vi "RT Main.vi"() -> ()   [LabVIEW 2023]
uses:
  <vilib>/Platform/TimedLoop/XDataNode/timing_clust.ctl
  <vilib>/Platform/TimedLoop/XDataNode/nitl_modes.ctl
  <vilib>/Platform/TimedLoop/XDataNode/wakeup.ctl
  <vilib>/DAQmx/read.llb/DAQmx Read (Analog 1D DBL NChan 1Samp).vi
  <vilib>/DAQmx/create/channels.llb/DAQmx Create Channel (AI-Position-LVDT).vi
  <vilib>/DAQmx/configure/timing.llb/DAQmx Timing (Sample Clock).vi
  <vilib>/DAQmx/miscellaneous.llb/DAQmx Fill In Error Info.vi
  <vilib>/platform/TimedLoop/XDataNode/XDataNode.xnode
  <vilib>/Platform/TimedLoop/XDataNode/XDNodeRunTimeDep.lvlib
panel:
  in  "Stop Button":bool
  in  "SCAS Controller Test Panel":enum32{"LVDT Test Page", "mA Output Test Page"}(tab)
  in  "Physical channels(PXI1Slot3/ai1:0)":tag="PXI1Slot3/ai1:0"
  in  "Voltage Excitation Value":dbl=3.0
  in  "Voltage excitation frequency":dbl=2050.0
  in  "Sensitivity":dbl=1.0
  in  "Samples per channel":i32=1000
  in  "Sample rate":dbl=1000.0 format="%0.2f"
  in  "Voltage excitation wire mode":i32(ring)=5 items=["4-Wire"=4, "5-Wire"=5, "6-Wire"=6]
  in  "Sample mode":i32(ring)=10123 items=["Finite Samples"=10178, "Continuous Samples"=10123, "Hardware Timed Single Point"=12522]
  in  "Sensivity value for calculation":dbl=1.0
  in  "Voltage excitation source":i32(ring)=10200 items=["Internal"=10200, "External"=10167, "None"=10230]
  in  "Sensitivity units":i32(ring)=12506 items=["mVolts/Volt/mMeter"=12506, "mVolts/Volt/0.001 Inch"=12505]
  in  "Units":i32(ring)=10219 items=["Meters"=10219, "Inches"=10379, "From Custom Scale"=10065]
  out "LVDT Output mm":dbl(graph)
  in  "resource name(PXI144::0::INSTR)":string="PXI144::0::INSTR"
  out "id string":string
  in  "Channel Output Number":u32=1
  in  "isolation switch":bool=TRUE
  in  "shorting switch":bool
  in  "Set Value mA":dbl(slide) scale=-24.0..24.0
  out "Get Value mA":dbl
  out "attr mode":u32
  out "error out":errorcluster
  # "Note1: Change Sensivity for adjusting the LVDT Output mm. 4340 reads the LVDT sensor mVolts/Volt/meter."
  # "Note2: Change Sensivity value for calculation if the sensivity is not enough to calculate LVDT Output mm"
  # "Note3: DONT assign 0 value for sensivity and sensivity value for calculation"
  # "Check the pickering card id"
  # "Check the Attr Mode is 3. 3 represents the -24 / +24 mA curret output mode."
  # "Check the isolation switch is \"CLOSE\"(1).(The button default state is \"OPEN\" inside pickering board)"
  # "Check the shorting switch is \"OPEN\"(0).(The button default state is \"OPEN\" inside pickering board)"
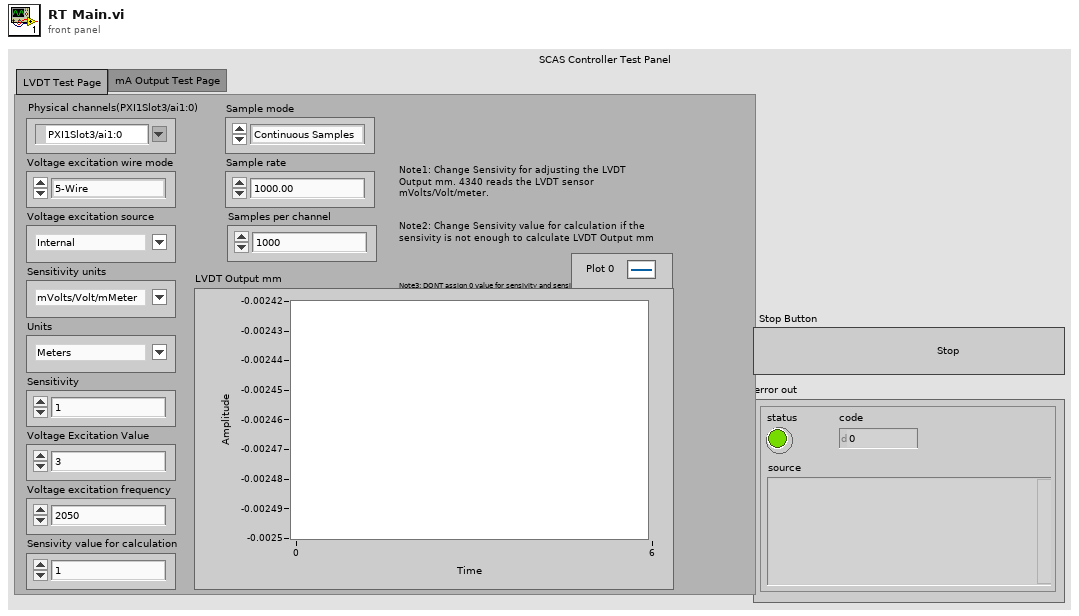
[diagram p1: front panel]
types:
  T1 = typedef "XDNodeRunTimeDep.lvlib/timing_clust.ctl" = cluster{"Expected End [f-1]":u64, "Actual End [f-1]":u64, "Finished Late? [f-1]":bool, "Expected End [i-1]":u64, "Actual End [i-1]":u64, "Finished Late? [i-1]":bool, "Expected Start [i]":u64, "Actual Start [i]":u64, "Expected Start [f]":u64, "Actual Start [f]":u64, "Source Name":string, "Structure Name":string, "Period":i64, "Deadline":i64, "Offset":i64, "Start":i64, "Priority":i32, "Timeout":i32, "Mode":T2, "Wakeup Reason":T3, "Error":errorcluster, "Source Type":string, "Secondary Source Type":string, "Global End Time":u64, "Global Start Time":u64, "Frame Duration":u64, "Iteration Duration":u64, "Assigned CPU":i32, "I/O Scan Engine Mode":u32}
  T2 = typedef "XDNodeRunTimeDep.lvlib/nitl_modes.ctl" = enum32{"No Change", "Process missed periods, maintain original phase", "Discard missed periods, maintain original phase", "Process missed periods, ignore original phase", "Discard missed periods, ignore original phase"}
  T3 = typedef "XDNodeRunTimeDep.lvlib/wakeup.ctl" = enum32{"Normal", "Aborted", "Asynchronous wakeup", "Timing source error", "Timed loop error", "Timeout"}
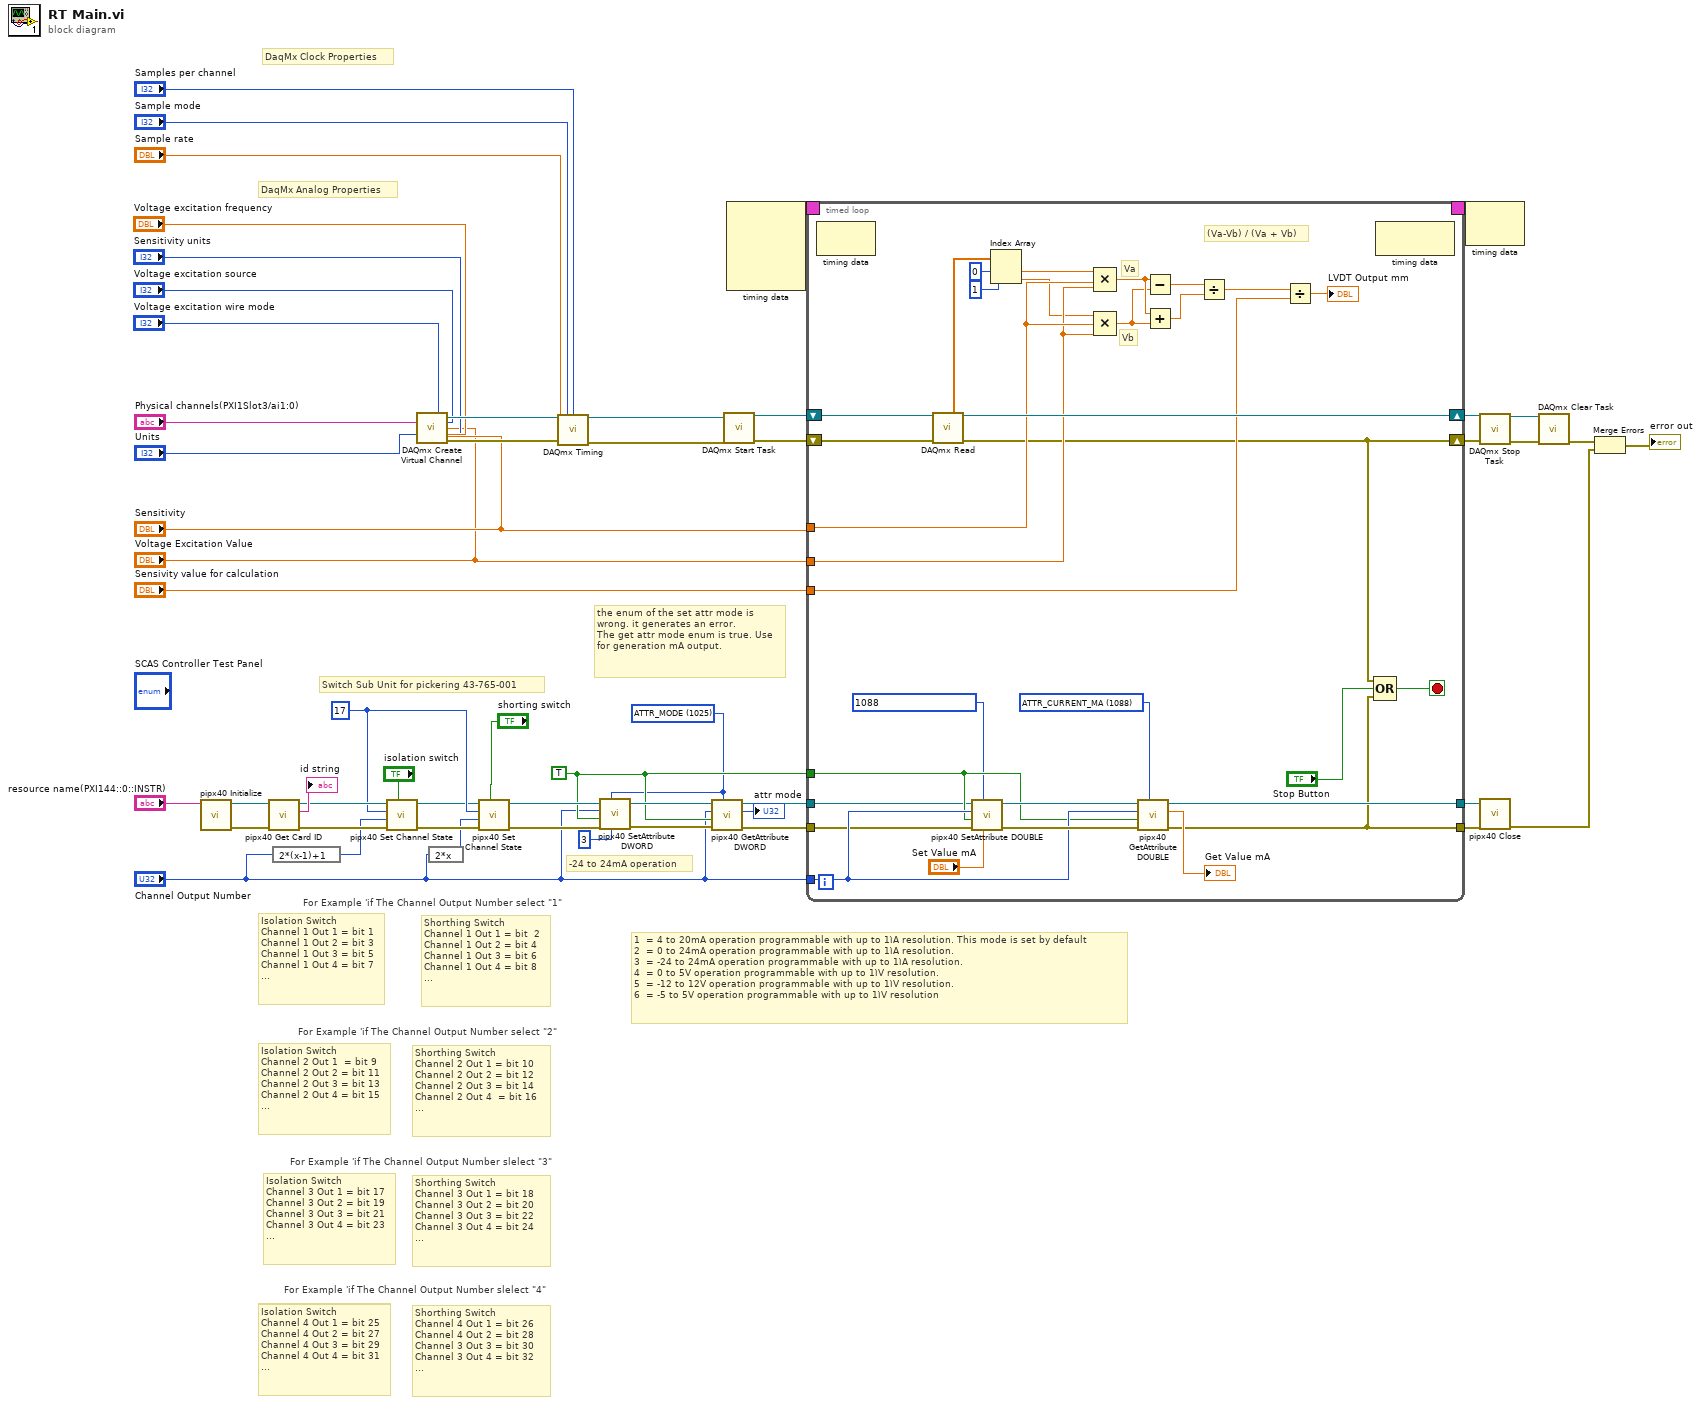
[diagram p0: block diagram]
diagram:
  w6 = u16 1025 items=["ATTR_TYPE"=1024, "ATTR_MODE"=1025, "ATTR_TS_SET_RANGE"=1034, "ATTR_VDT_AUTO_INPUT_ATTEN"=1104, "ATTR_VDT_ABS_POSITION"=1105, "ATTR_VDT_ABS_POSITION_B"=1106, "ATTR_VDT_OUT_GAIN   "=1111, "ATTR_VDT_MANUAL_INPUT_ATTEN"=1112, "ATTR_VDT_MODE"=1113, "ATTR_VDT_DELAY_A"=1114, "ATTR_VDT_DELAY_B"=1115, "ATTR_VDT_INPUT_LEVEL"=1116, "ATTR_VDT_INPUT_FREQ "=1117, "ATTR_VDT_OUT_LEVEL"=1118, "ATTR_VDT_DSPIC_VERSION  "=1119, "ATTR_VDT_INVERT_A"=1120, "ATTR_VDT_INVERT_B"=1121, "ATTR_VDT_LOS_THRESHOLD"=1125, "ATTR_VDT_SMPL_BUFFER_SIZE"=1126, "ATTR_LOAD"=1154, "ATTR_DIO_EXT_CLOCK_MODE"=1169, "ATTR_DIO_PATTERN_OFFSET"=1171, "ATTR_DIO_PATTERN_TOTAL_COUNT"=1172, "ATTR_C_DIO_START_POSITION"=4098, "ATTR_C_DIO_END_POSITION"=4099, "ATTR_C_DIO_ALL_PORT_DATA_OFFSET"=4107, "ATTR_C_DIO_FIFO_POS"=4108, "ATTR_C_CAPABILITIES"=4352, "ATTR_C_TEMP_SENSOR_COUNT"=4354, "ATTR_C_GA_SLOT_ADDRESS"=4355] ("Attribute Code")
  w8 = TRUE ("Is output")
  w23 = u32 17 ("subunit number")
  # "Isolation Switch\nChannel 4 Out 1 = bit 25\nChannel 4 Out 2 = bit 27\nChannel 4 Out 3 = bit 29\nChannel 4 Out 4 = bit 31\n..."
  # "For Example 'if The Channel Output Number slelect \"4\""
  # "Shorthing Switch\nChannel 4 Out 1 = bit 26  \nChannel 4 Out 2 = bit 28\nChannel 3 Out 3 = bit 30\nChannel 3 Out 4 = bit 32\n..."
  # "Isolation Switch\nChannel 4 Out 1 = bit 25\nChannel 4 Out 2 = bit 27\nChannel 4 Out 3 = bit 29\nChannel 4 Out 4 = bit 31\n..."
  # "For Example 'if The Channel Output Number slelect \"3\""
  # "Shorthing Switch\nChannel 3 Out 1 = bit 18  \nChannel 3 Out 2 = bit 20\nChannel 3 Out 3 = bit 22\nChannel 3 Out 4 = bit 24\n..."
  # "Isolation Switch\nChannel 3 Out 1 = bit 17\nChannel 3 Out 2 = bit 19\nChannel 3 Out 3 = bit 21\nChannel 3 Out 4 = bit 23\n..."
  # "For Example 'if The Channel Output Number select \"2\""
  # "Shorthing Switch\nChannel 2 Out 1 = bit 10  \nChannel 2 Out 2 = bit 12\nChannel 2 Out 3 = bit 14\nChannel 2 Out 4  = bit 16\n..."
  # "Isolation Switch\nChannel 2 Out 1  = bit 9\nChannel 2 Out 2 = bit 11\nChannel 2 Out 3 = bit 13\nChannel 2 Out 4 = bit 15\n..."
  # "For Example 'if The Channel Output Number select \"1\""
  # "the enum of the set attr mode is wrong. it generates an error. \nThe get attr mode enum is true. Use for generation mA output."
  # "DaqMx Analog Properties"
  # "DaqMx Clock Properties"
  # "-24 to 24mA operation"
  # "1  = 4 to 20mA operation programmable with up to 1ìA resolution. This mode is set by default\n2  = 0 to 24mA operation programmable with up to 1ìA resolution.\n3  = -24 to 24mA operation programmable with up to 1ìA resolution.\n4  = 0 to 5V operation programmable with up to 1ìV resolution.\n5  = -12 to 12V operation programmable with up to 1ìV resolution.\n6  = -5 to 5V operation programmable with up to 1ìV resolution"
  # "Shorthing Switch\nChannel 1 Out 1 = bit  2\nChannel 1 Out 2 = bit 4\nChannel 1 Out 3 = bit 6\nChannel 1 Out 4 = bit 8\n..."
  # "Isolation Switch\nChannel 1 Out 1 = bit 1\nChannel 1 Out 2 = bit 3\nChannel 1 Out 3 = bit 5\nChannel 1 Out 4 = bit 7\n..."
  # "Switch Sub Unit for pickering 43-765-001"
  n1 = call <instrlib>:"pipx40 Initialize.vi"("resource name"="resource name(PXI144::0::INSTR)") -> ("error out"=w30:errorcluster, "instrument handle out"=w26:refnum<visa-resource-name>)  [unwired: 9 in]
  n2 = call <instrlib>:"pipx40 Get Card ID.vi"("error in (no error)"=w30, "instrument handle"=w26) -> ("error out"=w29:errorcluster, "id string"=→"id string":string, "instrument handle out"=w24:refnum<visa-resource-name>)  [unwired: 7 in]
  n3 = expression code="2*(x-1)+1"("Channel Output Number") -> (w4:u32)
  n4 = call <instrlib>:"pipx40 Set Channel State.vi"("action"="isolation switch", "error in (no error)"=w29, "channel number"=w4, "subunit number"=w23, "instrument handle"=w24) -> ("error out"=w28:errorcluster, "instrument handle out"=w22:refnum<visa-resource-name>)  [unwired: 5 in]
  n5 = call-poly <vilib>:"DAQmx Create Virtual Channel.vi"("voltage excitation wire mode"="Voltage excitation wire mode", "physical channels"="Physical channels(PXI1Slot3/ai1:0)", "voltage excitation source"="Voltage excitation source", "voltage excitation value"="Voltage Excitation Value", "units"="Units", "voltage excitation frequency"="Voltage excitation frequency", "sensitivity"="Sensitivity", "sensitivity units"="Sensitivity units") -> ("task out"=w52:refnum<k21>, "error out"=w50:errorcluster)  [unwired: 6 in]
  n6 = expression code="2*x"("Channel Output Number") -> (w2:u32)
  n7 = call <instrlib>:"pipx40 Set Channel State.vi"("action"="shorting switch", "error in (no error)"=w28, "channel number"=w2, "subunit number"=w23, "instrument handle"=w22) -> ("error out"=w11:errorcluster, "instrument handle out"=w12:refnum<visa-resource-name>)  [unwired: 5 in]
  n8 = call-poly <vilib>:"DAQmx Timing.vi"("task/channels in"=w52, "sample mode"="Sample mode", "samples per channel"="Samples per channel", "rate"="Sample rate", "error in"=w50) -> ("task out"=w49:refnum<k21>, "error out"=w48:errorcluster)  [unwired: 9 in]
  n9 = call <instrlib>:"pipx40 SetAttribute DWORD.vi"("Value"=u32 3, "Attribute Code"=w6, "error in (no error)"=w11, "Is output"=w8, "Subunit"="Channel Output Number", "instrument handle"=w12) -> ("error out"=w10:errorcluster, "instrument handle out"=w9:refnum<visa-resource-name>)  [unwired: 4 in]
  n10 = call <instrlib>:"pipx40 GetAttribute DWORD.vi"("Attribute Code"=w6, "error in (no error)"=w10, "Is output"=w8, "Subunit"="Channel Output Number", "instrument handle"=w9) -> ("error out"=w15:errorcluster, "Value"=→"attr mode":u32, "instrument handle out"=w14:refnum<visa-resource-name>)  [unwired: 4 in]
  n11 = call <vilib>:"DAQmx Start Task.vi"("task/channels in"=w49, "error in"=w48) -> ("task out"=w45:refnum<k21>, "error out"=w44:errorcluster)  [unwired: 12 in]
  n12 = node-c288() -> (w37:T1)  [unwired: 4 in]
  n13 = timed-loop {
    timing: w37 -> [_]
    timing-out: [_] -> w36
    shift-right: [w83] -> w43
    shift-left: w45 -> [w85]
    shift-right: [w59] -> w42
    shift-left: w44 -> [w84]
    tunnel: "Sensitivity" -> [w79]
    tunnel: "Voltage Excitation Value" -> [w78]
    tunnel: "Sensivity value for calculation" -> [w72]
    tunnel: [w60] -> w20
    tunnel: [w66] -> w19
    tunnel: "Channel Output Number" -> [w63]
    tunnel: w8 -> [w62]
    tunnel: w14 -> [w58]
    tunnel: w15 -> [w57]
    stop <- w55 stop-if-true
    w56 = u16 1088 items=["ATTR_CURRENT_A"=1028, "ATTR_TS_LOW_RANGE_MIN"=1035, "ATTR_TS_LOW_RANGE_MED"=1036, "ATTR_TS_LOW_RANGE_MAX"=1037, "ATTR_TS_LOW_RANGE_MAX_DEV"=1038, "ATTR_TS_LOW_RANGE_PREC_PC"=1039, "ATTR_TS_LOW_RANGE_PREC_DELTA"=1040, "ATTR_TS_MED_RANGE_MIN"=1041, "ATTR_TS_MED_RANGE_MED"=1042, "ATTR_TS_MED_RANGE_MAX"=1043, "ATTR_TS_MED_RANGE_MAX_DEV"=1044, "ATTR_TS_MED_RANGE_PREC_PC"=1045, "ATTR_TS_MED_RANGE_PREC_DELTA"=1046, "ATTR_TS_HIGH_RANGE_MIN"=1047, "ATTR_TS_HIGH_RANGE_MED"=1048, "ATTR_TS_HIGH_RANGE_MAX"=1049, "ATTR_TS_HIGH_RANGE_MAX_DEV"=1050, "ATTR_TS_HIGH_RANGE_PREC_PC"=1051, "ATTR_TS_HIGH_RANGE_PREC_DELTA"=1052, "ATTR_CURRENT_MA"=1088, "ATTR_VOLTAGE_V"=1089, "ATTR_VOLTAGE_VAL "=1092, "ATTR_VDT_PERCENT_POSITION"=1107, "ATTR_VDT_PERCENT_POSITION_B"=1108, "ATTR_VDT_VOLTAGE_SUM"=1109, "ATTR_VDT_VOLTAGE_DIFF"=1110, "ATTR_VDT_INPUT_FREQ_HI_RES"=1124, "ATTR_VDT_MAX_OUT_VOLTAGE"=1129, " ATTR_VDT_MIN_OUT_VOLTAGE"=1130, "ATTR_VDT_MAX_IN_VOLTAGE"=1131, "ATTR_VDT_MIN_IN_VOLTAGE"=1132, "ATTR_VDT_PHASE_DELAY_A"=1133, "ATTR_VDT_PHASE_DELAY_B"=1134, "ATTR_RESOLVER_ROTATE_SPEED"=1138, "ATTR_RESOLVER_POSITION"=1139, "ATTR_RESOLVER_POSITION_0_360"=1140, "ATTR_RAMP_RESPONSE"=1142, "ATTR_C_DIO_INT_CLOCK_FREQ"=4097, "ATTR_C_DIO_CLOCK_DELAY"=4114] ("Attribute Code")
    # "(Va-Vb) / (Va + Vb)"
    # "Vb"
    # "Va"
    n14 = node-c288() -> ()  [unwired: 1 in, 1 out]
    n15 = call-poly <vilib>:"DAQmx Read.vi"("task/channels in"=w85, "error in"=w84) -> ("task out"=w83:refnum<k21>, "data"=w82:dbl[], "error out"=w59:errorcluster)  [unwired: 11 in]
    n16 = call <instrlib>:"pipx40 SetAttribute DOUBLE.vi"("Value"="Set Value mA", "Attribute Code"=u32 1088, "error in (no error)"=w57, "Is output"=w62, "Subunit"=w63, "instrument handle"=w58) -> ("error out"=w68:errorcluster, "instrument handle out"=w67:refnum<visa-resource-name>)  [unwired: 4 in]
    n17 = Index Array(array=w82, index #1=0 ("index"), index #2=1 ("index")) -> (element #1=w76:dbl, element #2=w77:dbl)
    n18 = Compound Arithmetic op=MULTIPLY(w76, w79, w78) -> (w70:dbl)
    n19 = Compound Arithmetic op=MULTIPLY(w77, w79, w78) -> (w69:dbl)
    n20 = call <instrlib>:"pipx40 GetAttribute DOUBLE.vi"("Attribute Code"=w56, "error in (no error)"=w68, "Is output"=w62, "Subunit"=w63, "instrument handle"=w67) -> ("error out"=w60:errorcluster, "Value"=→"Get Value mA":dbl, "instrument handle out"=w66:refnum<visa-resource-name>)  [unwired: 4 in]
    n21 = Subtract(x=w70, y=w69) -> (x-y=w75:dbl)
    n22 = Add(x=w70, y=w69) -> (x+y=w74:dbl)
    n23 = Divide(x=w75, y=w74) -> (x/y=w73:dbl)
    n24 = Divide(x=w73, y=w72) -> (x/y=→"LVDT Output mm":dbl)
    n25 = Compound Arithmetic op=OR(w59, "Stop Button", w60) -> (w55:bool)
    n26 = node-c288() -> ()  [unwired: 1 in, 1 out]
  }
  n27 = node-c288(w36) -> ()  [unwired: 1 out]
  n28 = call <vilib>:"DAQmx Stop Task.vi"("task/channels in"=w43, "error in"=w42) -> ("task out"=w40:refnum<k21>, "error out"=w41:errorcluster)  [unwired: 12 in]
  n29 = call <instrlib>:"pipx40 Close.vi"("error in (no error)"=w20, "instrument handle"=w19) -> ("error out"=w16:errorcluster)  [unwired: 9 in]
  n30 = call <vilib>:"DAQmx Clear Task.vi"("task in"=w40, "error in"=w41) -> ("error out"=w17:errorcluster)  [unwired: 13 in]
  n31 = Merge Errors(w17, w16) -> (→"error out":errorcluster)
